vi "Record Call.vi"(10 "VI Call":refnum<class "VI Call.lvclass">, 11 "One Of In":refnum<class "At Least.lvclass">) -> (3 "One Of Out":refnum<class "At Least.lvclass">)   [LabVIEW 2020, in "At Least.lvlib" / "At Least.lvclass"]
uses:
  At Least.lvclass
  Core/VI Call/VI Call.lvclass
  At Least.lvclass/At Least.ctl
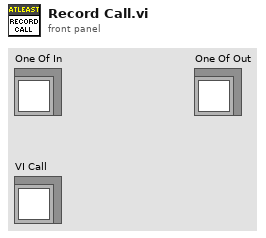
[diagram p1: front panel]
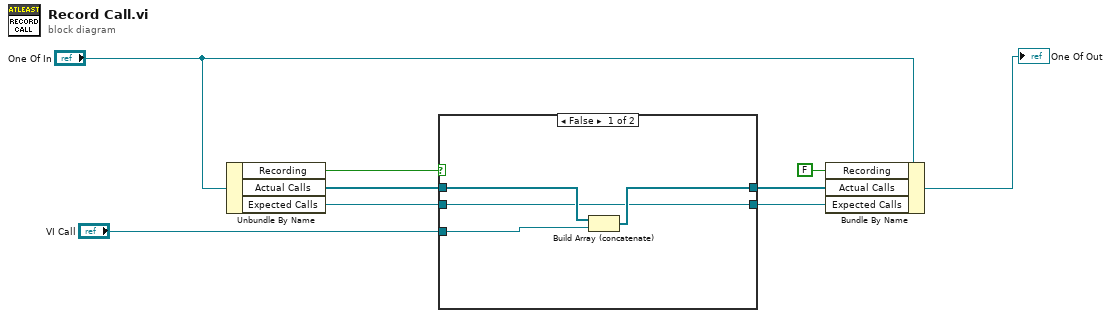
[diagram p0: block diagram]
diagram:
  n1 = Unbundle By Name("One Of In") -> ("Recording"=w5:bool, "Actual Calls"=w9:refnum<class "VI Call.lvclass">[], "Expected Calls"=w3:refnum<class "VI Call.lvclass">)
  n2 = case shown="False" w5 {
    tunnel: w9 -> [w13 w15]
    tunnel: [w12 w15] -> w8
    tunnel: "VI Call" -> [w10 w14]
    tunnel: w3 -> [w11 _]
    tunnel: [w11 w14] -> w1
    frame False {
      n3 = Build Array (concatenate)(w13, w10) -> (w12:refnum<class "VI Call.lvclass">[])
    }
    frame True {
    }
  }
  n4 = Bundle By Name(cluster="One Of In", "Recording"=FALSE, "Actual Calls"=w8, "Expected Calls"=w1) -> (→"One Of Out":refnum<class "At Least.lvclass">)
